vi "XYM单元件读写.vi"(8 "错误输入":errorcluster, 9 "Read？":bool, 10 "Component Assemble Input":T1, 11 "引用":refnum<k7>) -> (0 "错误输出":errorcluster, 2 "Read State":bool, 3 "引用输出":refnum<k7>)   [LabVIEW 2017]
uses:
  Component Assemble Input.ctl
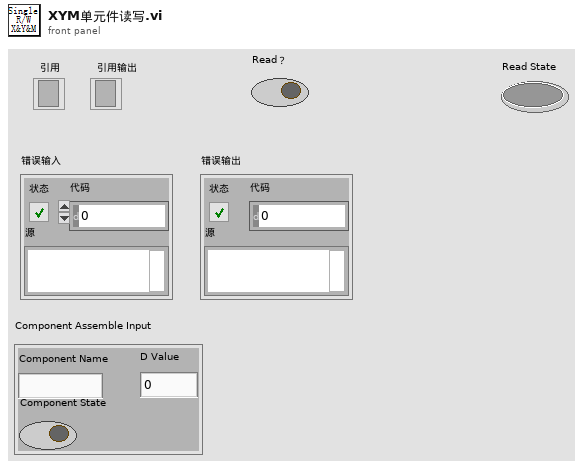
[diagram p1: front panel]
types:
  T1 = typedef "Component Assemble Input.ctl" = cluster{"Component Name":string, "Component State":bool, "D Value":i32}
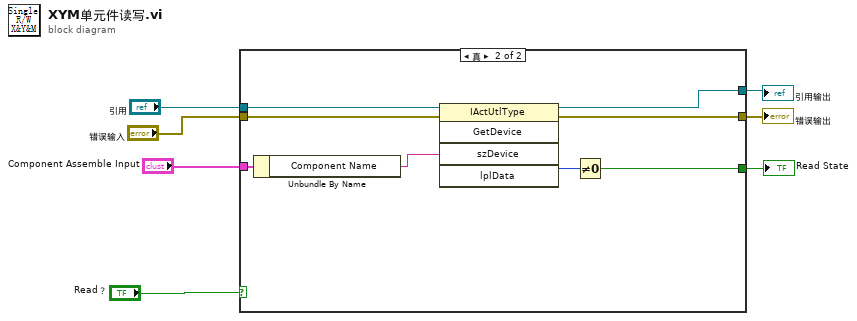
[diagram p0: block diagram]
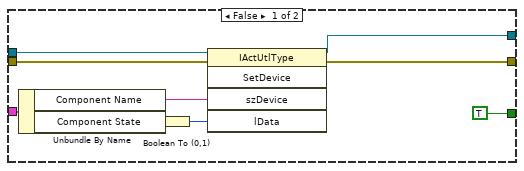
[diagram p2: hidden frame]
diagram:
  n1 = case shown="真" "Read？" {
    tunnel: "引用" -> [w16 w24]
    tunnel: [w10 w23] -> w6
    tunnel: "错误输入" -> [w15 w22]
    tunnel: [w9 w21] -> w4
    tunnel: "Component Assemble Input" -> [w14 w20]
    tunnel: [TRUE w17] -> w1
    frame False {
      n2 = Unbundle By Name(w14) -> ("Component Name"=w11:string, "Component State"=w13:bool)
      n3 = Boolean To (0,1)(Boolean=w13) -> (0, 1=w12:i16)
      n4 = invoke on="调用节点" class="IActUtlType" method="SetDevice"(reference=w16, error in=w15, "szDevice"=w11, "lData"=w12) -> (reference out=w10:refnum<k7>, error out=w9:errorcluster)  [unwired: 1 in, 3 out]
    }
    frame True {
      n5 = Unbundle By Name(w20) -> ("Component Name"=w19:string)
      n6 = invoke on="调用节点" class="IActUtlType" method="GetDevice"(reference=w24, error in=w22, "szDevice"=w19) -> (reference out=w23:refnum<k7>, error out=w21:errorcluster, "lplData"=w18:i32)  [unwired: 2 in, 2 out]
      n7 = Not Equal To 0?(x=w18) -> (x != 0?=w17:bool)
    }
  }
  "引用输出" <- w6
  "错误输出" <- w4
  "Read State" <- w1
